vi "_Check_If_Error.vi"(8 "error in (no error)":errorcluster, 11 "Postgres Connector In":refnum<class "Postgres Connector.lvclass">) -> (0 "error out":errorcluster, 3 "Postgres Connector In 2":refnum<class "Postgres Connector.lvclass">)   [LabVIEW 2019, in "PG_LIB.lvlib" / "Postgres Connector.lvclass"]
uses:
  Postgres Connector.lvclass
  Cluster_Reader_Infos.ctl
  Enum_RowDescription_State_Machine.ctl
  Postgres Connector.lvclass/Postgres Connector.ctl
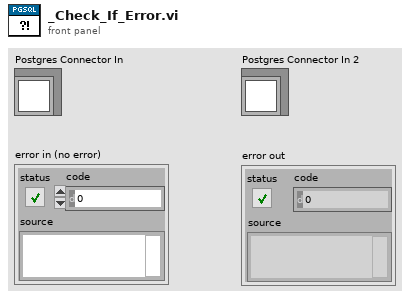
[diagram p1: front panel]
types:
  T1 = typedef "PG_LIB.lvlib/Postgres Connector.lvclass/Enum_RowDescription_State_Machine.ctl" = enum16{"Check For Error", "Wait For T", "Wait For D", "Wait For Z", "C Byte Length", "Z Byte Length", "n Byte Length", "Byte Length", "Get Infos", "Check For End", "Flush", "Quit"}
  T2 = typedef "PG_LIB.lvlib/Postgres Connector.lvclass/Cluster_Reader_Infos.ctl" = cluster{"Byte Length":i32}
  T3 = enum16{"Standard", "Buffered", "CRLF", "Immediate"}
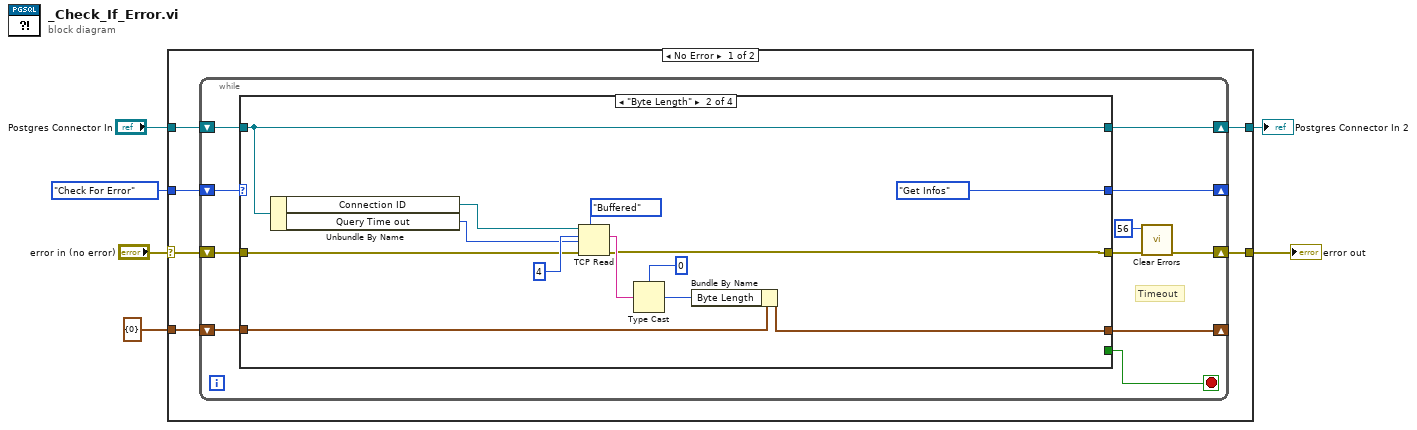
[diagram p0: block diagram]
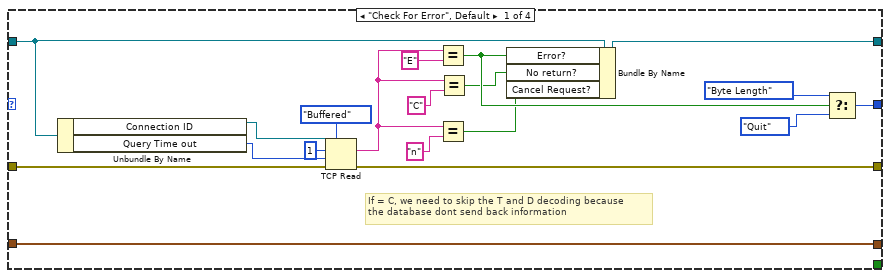
[diagram p2: hidden frame]
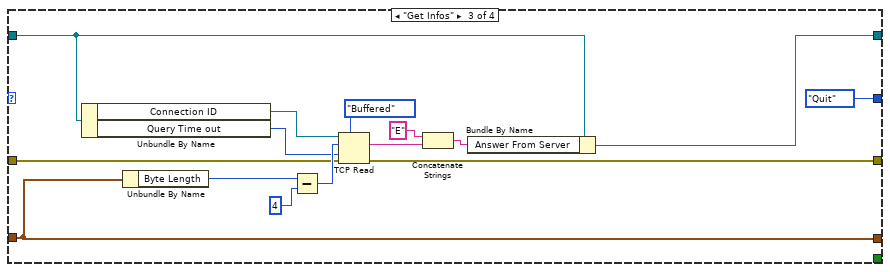
[diagram p3: hidden frame]
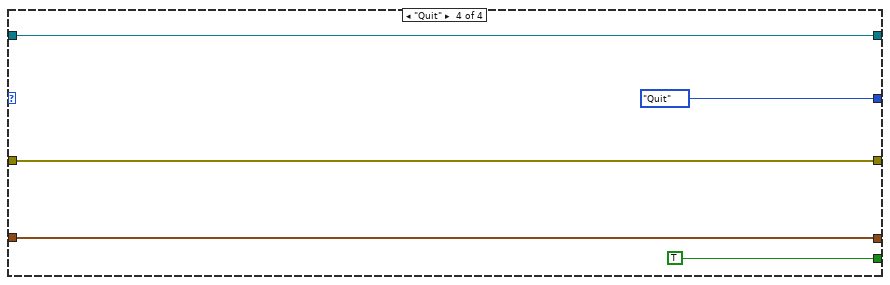
[diagram p4: hidden frame]
diagram:
  n1 = case shown="No Error" "error in (no error)" {
    selector: "error in (no error)" -> [w12 w77]
    tunnel: "Postgres Connector In" -> [w7 w76]
    tunnel: Enum_RowDescription_State_Machine."Check For Error" -> [w11 _]
    tunnel: [w10 w77] -> w4
    tunnel: T2 {"Byte Length"=0} ("Reader_Infos") -> [w9 _]
    tunnel: [w8 w76] -> w1
    frame No Error {
      n2 = while {
        shift-right: [w20] -> w10
        shift-left: w12 -> [w23]
        shift-right: [w18] -> _
        shift-left: w11 -> [w22]
        shift-right: [w16] -> _
        shift-left: w9 -> [w17]
        shift-right: [w14] -> w8
        shift-left: w7 -> [w13]
        stop <- w15 stop-if-true
        # "Timeout"
        n3 = case shown="\"Byte Length\"" w22 {
          tunnel: w23 -> [w39 w49 w66 w74]
          tunnel: [w38 w46 w65 w74] -> w21
          tunnel: [w34 Enum_RowDescription_State_Machine."Get Infos" Enum_RowDescription_State_Machine."Quit" Enum_RowDescription_State_Machine."Quit"] -> w18
          tunnel: w17 -> [w37 w48 w63 w75]
          tunnel: [w37 w47 w63 w75] -> w16
          tunnel: [_ _ _ TRUE] -> w15
          tunnel: [w31 w44 w60 w71] -> w14
          tunnel: w13 -> [w30 w44 w61 w71]
          frame "Check For Error", Default {
            # "If = C, we need to skip the T and D decoding because \nthe database dont send back information"
            n4 = Unbundle By Name(w30) -> ("Connection ID"=w41:refnum<k5>, "Query Time out"=w27:i32)
            n5 = TCP Read(connection ID=w41, bytes to read=1, error in (no error)=w39, 7:T3."Buffered" ("mode (standard)"), 9:w27) -> (data out=w25:string, error out=w38:errorcluster)  [unwired: 1 out]
            n6 = Equal?(x=w25, y="E") -> (x = y?=w32:bool)
            n7 = Equal?(x=w25, y="n") -> (x = y?=w24:bool)
            n8 = Equal?(x=w25, y="C") -> (x = y?=w28:bool)
            n9 = Bundle By Name(cluster=w30, "Error?"=w32, "No return?"=w28, "Cancel Request?"=w24) -> (w31:refnum<class "Postgres Connector.lvclass">)
            n10 = Select(t=Enum_RowDescription_State_Machine."Byte Length", s=w32, f=Enum_RowDescription_State_Machine."Quit") -> (s? t:f=w34:T1)
          }
          frame "Byte Length" {
            n11 = Unbundle By Name(w44) -> ("Connection ID"=w55:refnum<k5>, "Query Time out"=w43:i32)
            n12 = TCP Read(connection ID=w55, bytes to read=4, error in (no error)=w49, 7:T3."Buffered" ("mode (standard)"), 9:w43) -> (data out=w54:string, error out=w46:errorcluster)  [unwired: 1 out]
            n13 = Type Cast(type=0, x=w54) -> (*(type *) &x=w53:i32)
            n14 = Bundle By Name(cluster=w48, "Byte Length"=w53) -> (w47:T2)
          }
          frame "Get Infos" {
            n15 = Unbundle By Name(w61) -> ("Connection ID"=w62:refnum<k5>, "Query Time out"=w56:i32)
            n16 = Unbundle By Name(w63) -> ("Byte Length"=w68:i32)
            n17 = Subtract(x=w68, y=4 ("bytes to read")) -> (x-y=w67:i32)
            n18 = TCP Read(connection ID=w62, bytes to read=w67, error in (no error)=w66, 7:T3."Buffered" ("mode (standard)"), 9:w56) -> (data out=w59:string, error out=w65:errorcluster)  [unwired: 1 out]
            n19 = Concatenate Strings("E" ("string"), w59) -> (w58:string)
            n20 = Bundle By Name(cluster=w61, "Answer From Server"=w58) -> (w60:refnum<class "Postgres Connector.lvclass">)
          }
          frame "Quit" {
          }
        }
        n21 = call <vilib>:"Clear Errors.vi"("error in (no error)"=w21, "specific error code to clear (0: all)"=56) -> ("error out"=w20:errorcluster)  [unwired: 4 in, 1 out]
      }
    }
    frame Error {
    }
  }
  "error out" <- w4
  "Postgres Connector In 2" <- w1
